vi "Read Meta Data.vi"(11 "Tree Data In":refnum<class "Tree Data.lvclass">) -> (1 "Meta Data":string, 3 "Tree Data Out":refnum<class "Tree Data.lvclass">)   [LabVIEW 2017, in "Tree API.lvlib" / "Tree Data.lvclass"]
doc: "Write the Meta Data associated with this Tree Data type. This can store any information."
uses:
  Tree Data.lvclass
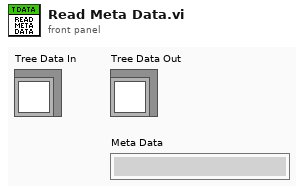
[diagram p1: front panel]
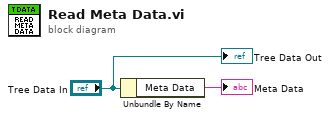
[diagram p0: block diagram]
diagram:
  n1 = Unbundle By Name("Tree Data In") -> ("Meta Data"=→"Meta Data":string)
  "Tree Data Out" <- "Tree Data In"
